vi "子界面2.vi"(10 "用户事件输出":refnum<user-event>, 11 "子面板":refnum<vi>) -> ()   [LabVIEW 2012]
panel:
  in  "退出":bool caption="停止"
  # "这是子面板2"
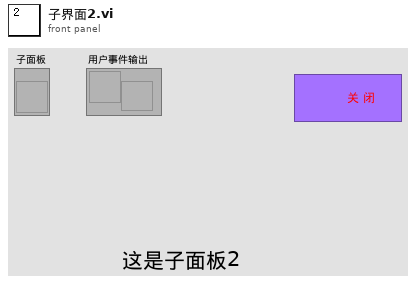
[diagram p1: front panel]
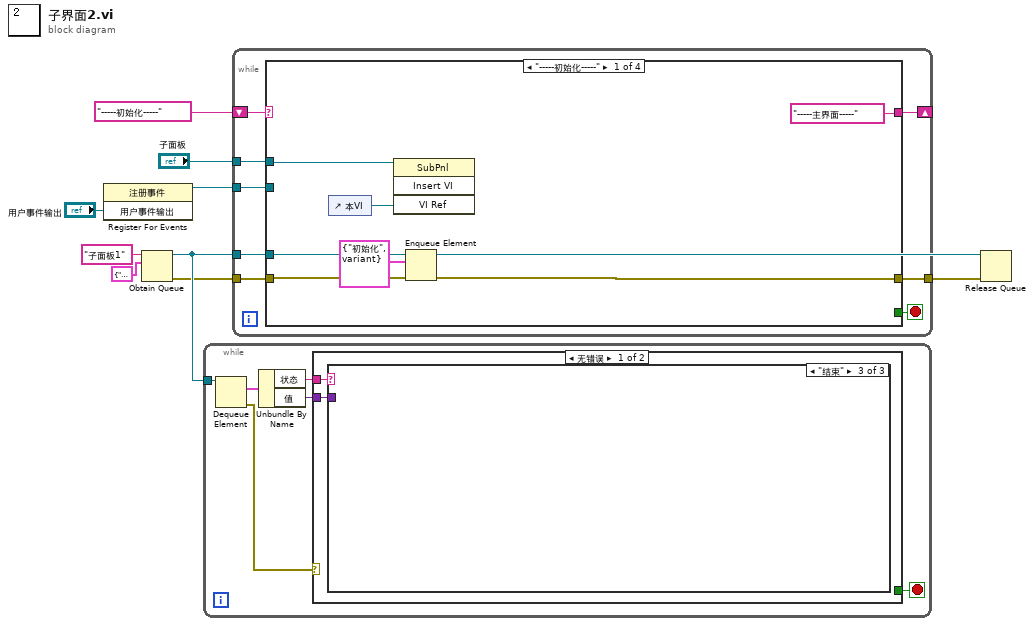
[diagram p0: block diagram]
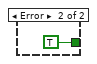
[diagram p4: hidden frame]
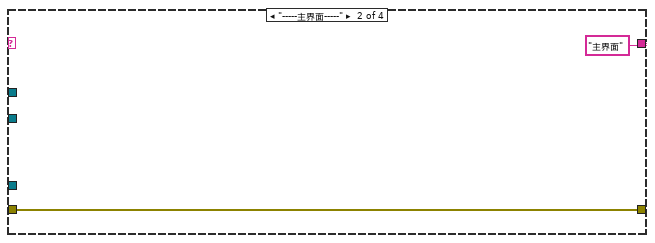
[diagram p5: hidden frame]
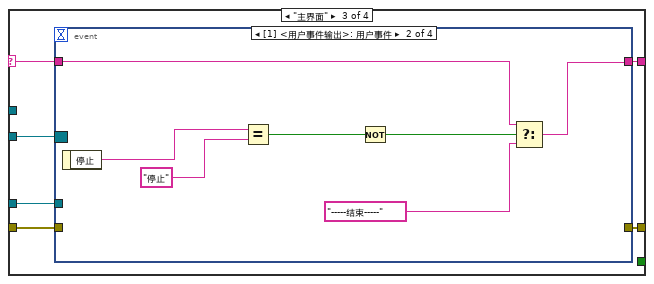
[diagram p6: hidden frame]
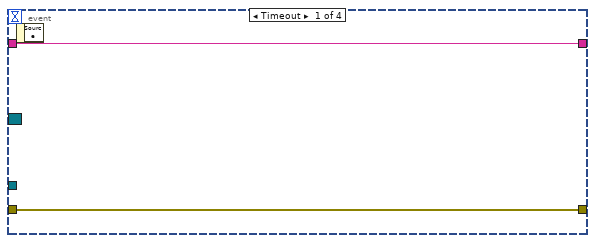
[diagram p7: hidden frame]
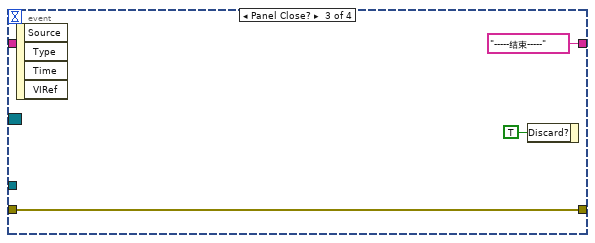
[diagram p8: hidden frame]
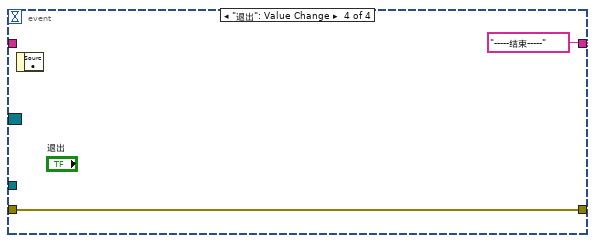
[diagram p9: hidden frame]
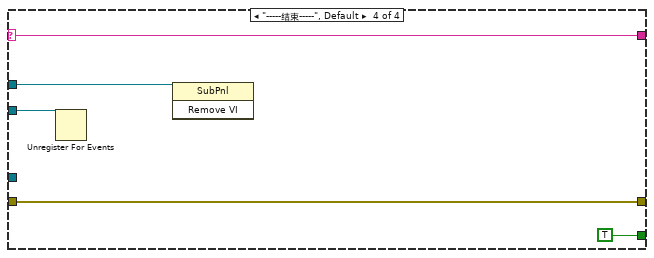
[diagram p10: hidden frame]
diagram:
  n1 = register-events("用户事件输出") -> (reference out=w1:refnum<event-registration>)  [unwired: 2 in, 1 out]
  n2 = Obtain Queue(name (unnamed)="子面板1" ("名称（未命名）"), element data type=cluster{"状态":string, "值":variant} {"状态"="", "值"=variant} ("队列元素")) -> (queue out=w9:refnum<queue>, error out=w7:errorcluster)  [unwired: 3 in, 1 out]
  n3 = while {
    tunnel: w9 -> [w15]
    stop <- w13 stop-if-true
    n4 = Dequeue Element(queue=w15) -> (element=w12:cluster{"状态":string, "值":variant}, error out=w14:errorcluster)  [unwired: 2 in, 2 out]
    n5 = Unbundle By Name(w12) -> ("状态"=w11:string, "值"=w10:variant)
    n6 = case shown="无错误" w14 {
      tunnel: [_ TRUE] -> w13
      tunnel: w11 -> [w17 _]
      tunnel: w10 -> [w16 _]
      frame No Error {
        n7 = case shown="\"结束\"" w17 {
          tunnel: w16 -> [_ _ _]
          frame "假", Default {
          }
          frame "初始化" {
          }
          frame "结束" {
          }
        }
      }
      frame Error {
      }
    }
  }
  n8 = while {
    tunnel: w9 -> [w26]
    shift-right: [w25] -> _
    shift-left: "-----初始化-----" -> [w24]
    tunnel: w7 -> [w22]
    tunnel: [w21] -> w6
    tunnel: "子面板" -> [w19]
    tunnel: w1 -> [w20]
    stop <- w23 stop-if-true
    n9 = case shown="\"-----初始化-----\"" w24 {
      selector: w24 -> [_ _ w37 w59]
      tunnel: w26 -> [w32 _ w41 _]
      tunnel: w22 -> [w31 w34 w40 w60]
      tunnel: [w27 w34 w39 w60] -> w21
      tunnel: ["-----主界面-----" "主界面" w38 w59] -> w25
      tunnel: [_ _ _ TRUE] -> w23
      tunnel: w20 -> [_ _ w36 w57]
      tunnel: w19 -> [w29 _ _ w56]
      frame "-----初始化-----" {
        n10 = control-ref of="本VI"() -> (w28:refnum<vi>)
        n11 = invoke class="SubPnl" method="Insert VI"(reference=w29, "VI Ref"=w28) -> ()  [unwired: 2 in, 4 out]
        n12 = Enqueue Element(queue=w32, element=cluster{"状态":string, "值":variant} {"状态"="初始化", "值"=variant} ("元素"), error in (no error)=w31) -> (error out=w27:errorcluster)  [unwired: 1 in, 2 out]
      }
      frame "-----主界面-----" {
      }
      frame "主界面" {
        n13 = event shown="[1] <用户事件输出>: 用户事件" {
          selector: w36 -> [_ _ _ _]
          dyn-events: _ -> [_ _ _ _]
          timeout: _ -> [_ _ _ _]
          tunnel: w41 -> [_ _ _ _]
          tunnel: w40 -> [w42 _ w52 w55]
          tunnel: [w42 _ w52 w55] -> w39
          tunnel: [w43 w46 "-----结束-----" "-----结束-----"] -> w38
          tunnel: w37 -> [w43 w47 _ _]
          event Timeout {
            n14 = event-data() -> ()  [unwired: 1 in, 1 out]
          }
          event User Event {
            n15 = event-data() -> ("停止"=w50:string)  [unwired: 1 in]
            n16 = Equal?(x=w50, y="停止") -> (x = y?=w45:bool)
            n17 = Not(x=w45) -> (.not. x?=w44:bool)
            n18 = Select(t=w47, s=w44, f="-----结束-----" ("真状态")) -> (s? t:f=w46:string)
          }
          event Panel Close? {
            n19 = event-data() -> ()  [unwired: 1 in, 4 out]
            n20 = event-data("Discard?"=TRUE ("放弃？")) -> ()  [unwired: 1 in, 1 out]
          }
          event "退出": Value Change {
            n21 = event-data() -> ()  [unwired: 1 in, 1 out]
          }
        }
      }
      frame "-----结束-----", Default {
        n22 = Unregister For Events(event registration refnum=w57) -> ()  [unwired: 1 in, 1 out]
        n23 = invoke class="SubPnl" method="Remove VI"(reference=w56) -> ()  [unwired: 2 in, 3 out]
      }
    }
  }
  n24 = Release Queue(queue=w9, error in (no error)=w6) -> ()  [unwired: 1 in, 3 out]
